vi "Sample-2.vi"() -> ()   [LabVIEW 2010]
panel:
  out "x .xor. y?":i32
  out "x+1":dbl
  out "XY Graph":cluster{"Y":dbl[], "Y":dbl[]}[](graph)
  out "x-y":i32[](array[numeric])
  out "offset past match":i32
  out "after substring":string
  out "match substring":string
  out "before substring":string
  out "Waveform Graph 2":i32[](graph)
  out "Array 2":i32[](array[numeric])
  out "Numeric 4":i32
  out "Numeric 3":i32
  out "Array":dbl[](array[numeric])
  out "element":i32
  out "Waveform Graph":i32[](graph)
  out "Numeric 2":i32
  out "Numeric":i32
  out "Boolean":bool
  out "size(s)":i32[](array[numeric])
  out "subarray":i32[](array[numeric])
  out "result string":string
  out "replaced substring":string
  out "output array":i32[](array[numeric])
  out "x*y":dbl
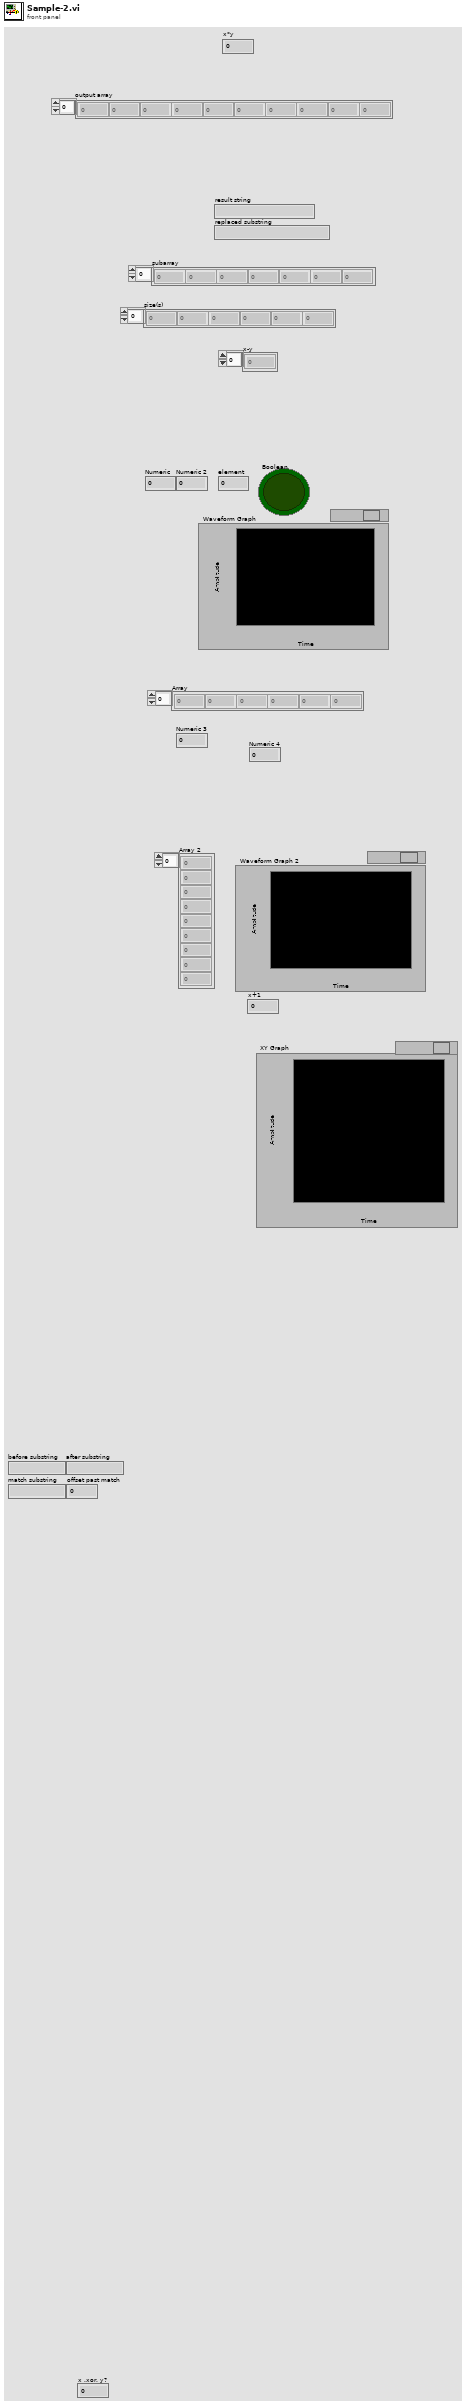
[diagram p1: front panel]
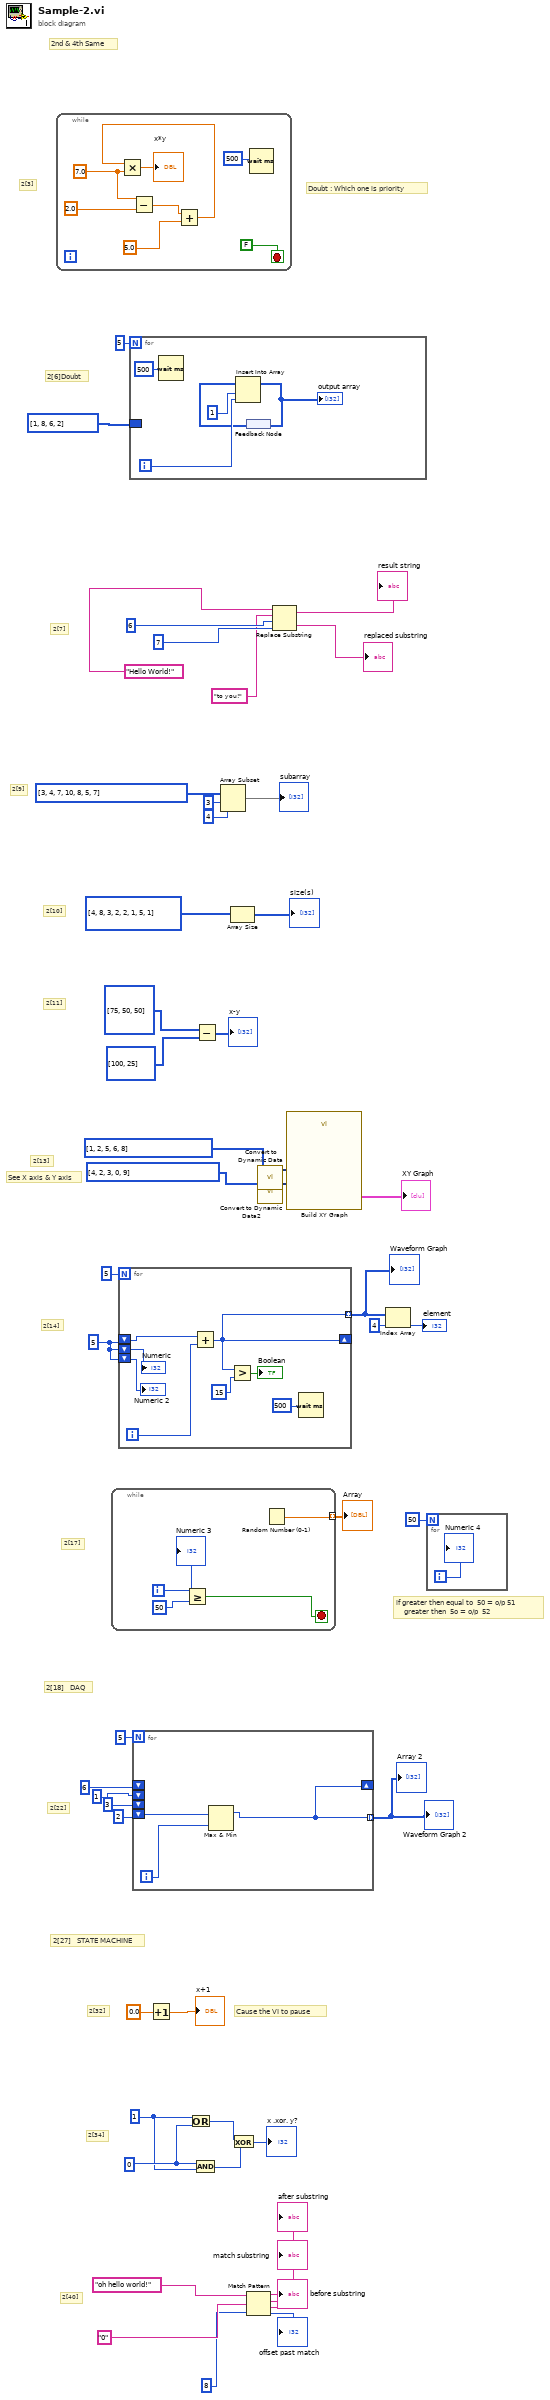
[diagram p0: block diagram]
diagram:
  w3 = 0
  w2 = 1
  w34 = 5
  # "See X axis & Y axis"
  # "2nd & 4th Same"
  # "2[34]"
  # "Cause the VI to pause"
  # "2[32]"
  # "2[27]   STATE MACHINE"
  # "2[18]   DAQ"
  # "2[13]"
  # "2[11]"
  # "2[40]"
  # "2[3]"
  # "Doubt : Which one is priority"
  # "2[22]"
  # "if greater then equal to  50 = o/p 51\n    greater then  5o = o/p  52"
  # "2[17]"
  # "2[14]"
  # "2[10]"
  # "2[9]"
  # "2[7]"
  # "2[6]Doubt"
  n1 = while {
    stop <- FALSE ("stop") stop-if-true
    w55 = 7.0 ("y")
    n2 = Subtract(x=w55, y=2.0) -> (x-y=w54:dbl)
    n3 = Add(x=w54, y=5.0) -> (x+y=w53:dbl)
    n4 = Multiply(x=w53, y=w55) -> (x*y=→"x*y":dbl)
    n5 = Wait (ms)(milliseconds to wait=u32 500 ("millisecond timer value")) -> ()  [unwired: 1 out]
  }
  n6 = while {
    tunnel: [w61] -> w30 mode=indexing
    i -> [w60]
    stop <- w58 stop-if-true
    n7 = Greater Or Equal?(x=w60, y=50) -> (x >= y?=w58:bool)
    n8 = Random Number (0-1)() -> (number: 0 to 1=w61:dbl)
    "Numeric 3" <- w60
  }
  "Array" <- w30
  n9 = for {
    N: 5 -> [_]
    shift-right: [w63] -> _
    shift-left: w34 -> [w66]
    shift-left: w34 -> [w65]
    shift-left: w34 -> [w64]
    tunnel: [w63] -> w32 mode=indexing
    i -> [w67]
    n10 = Add(x=w66, y=w67) -> (x+y=w63:i32)
    n11 = Greater?(x=w63, y=15) -> (0:→"Boolean":bool)
    n12 = Wait (ms)(milliseconds to wait=u32 500) -> ()  [unwired: 1 out]
    "Numeric" <- w65
    "Numeric 2" <- w64
  }
  "Waveform Graph" <- w32
  n13 = for {
    N: 5 -> [_]
    border: i32[] [1, 8, 6, 2] -> [_]
    i -> [w73]
    n14 = Wait (ms)(milliseconds to wait=u32 500 ("millisecond timer value")) -> ()  [unwired: 1 out]
    n15 = feedback #1() -> (w71:i32[])
    n16 = Insert Into Array "Insert Into Array"(array=w71, index=1, new element=w73) -> (w72:i32[])
    "output array" <- w72
    n17 = feedback-in #1(w72) -> ()
  }
  n18 = for {
    N: 5 -> [_]
    shift-right: [w75] -> _
    shift-left: 6 -> [_]
    shift-left: 1 -> [_]
    shift-left: 3 -> [_]
    shift-left: 2 -> [w77]
    tunnel: [w75] -> w23 mode=indexing
    i -> [w76]
    n19 = Max & Min(x=w77, y=w76) -> (max(x,y)=w75:i32)  [unwired: 1 out]
  }
  "Array 2" <- w23
  "Waveform Graph 2" <- w23
  n20 = Increment(x=0.0) -> (x+1=→"x+1":dbl)
  n21 = Or(x=w2, y=w3) -> (x .or. y?=w5:i32)
  n22 = And(x=w3, y=w2) -> (x .and. y?=w4:i32)
  n23 = Subtract(x=i32[] [75, 50, 50], y=i32[] [100, 25]) -> (x-y=→"x-y":i32[])
  n24 = Array Subset "Array Subset"(array=i32[] [3, 4, 7, 10, 8, 5, 7], index=3, length=4) -> (→"subarray":i32[])
  n25 = Array Size(array=i32[][] [[4, 8, 3, 2], [2, 1, 5, 1]]) -> (size(s)=→"size(s)":i32[])
  n26 = Exclusive Or(1:w4, 2:w5) -> (0:→"x .xor. y?":i32)
  n27 = Match Pattern(string="oh hello world!", regular expression="0", offset (0)=8) -> (before substring=→"before substring":string, match substring=→"match substring":string, after substring=→"after substring":string, offset past match=→"offset past match":i32)
  n28 = call "Convert to Dynamic Data"("Array"=i32[] [1, 2, 5, 6, 8]) -> ("Dynamic Data Type"=w10:dynamicdata)  [unwired: 3 in]
  n29 = call "Convert to Dynamic Data2"("Array"=i32[] [4, 2, 3, 0, 9]) -> ("Dynamic Data Type"=w8:dynamicdata)  [unwired: 3 in]
  n30 = Replace Substring(2:7 ("length (len. of substring)"), 3:6 ("offset (0)"), 4:"to you!" ("substring (\"\")"), 5:"Hello World!" ("string")) -> (0:→"replaced substring":string, 1:→"result string":string)
  n31 = call "Build XY Graph"("Y Input"=w8, "X Input"=w10) -> ("XY Graph"=→"XY Graph":cluster{"X":dbl[], "Y":dbl[]}[])  [unwired: 8 in, 1 out]
  n32 = Index Array "Index Array"(array=w32, index=4) -> (element=→"element":i32)
  n33 = for {
    N: 50 -> [_]
    i -> [w78]
    "Numeric 4" <- w78
  }
